vi "Test_peregrine_parameters.vi"() -> ()   [LabVIEW 2019]
panel:
  in  "Value\n(first motor write)":dbl
  out "Decoded value response\n(second motor read)":dbl
  out "Raw value response\n(second motor read)":i32
  out "Key response\n(second motor read)":u32
  out "Decoded value response\n(first motor write)":dbl
  out "Raw value response\n(first motor write)":i32
  out "Key response\n(first motor write)":u32
  out "Decoded value response\n(first motor read)":dbl
  out "Raw value response\n(first motor read)":i32
  out "Key response\n(first motor read)":u32
  in  "Select parameter\n(first motor write)":T1(ring)
  in  "Select parameter\n(first and second for motor read)":T1(ring)
  out "Value response\n(second read)":i32
  out "Key response\n(second read)":u32
  out "Value response\n(first write)":i32
  out "Key response\n(first write)":u32
  in  "Select parameter\n(first write)":T2(ring)
  out "Value response\n(first read)":i32
  out "Key response\n(first read)":u32
  in  "Select parameter\n(first and second read)":T3(ring)
  in  "Address":u8
  in  "COM Port for serial\nconnection. Check device\nmanager.":string
  # "Peregrine test program parameter set and read"
  # "General inputs"
  # "Inputs"
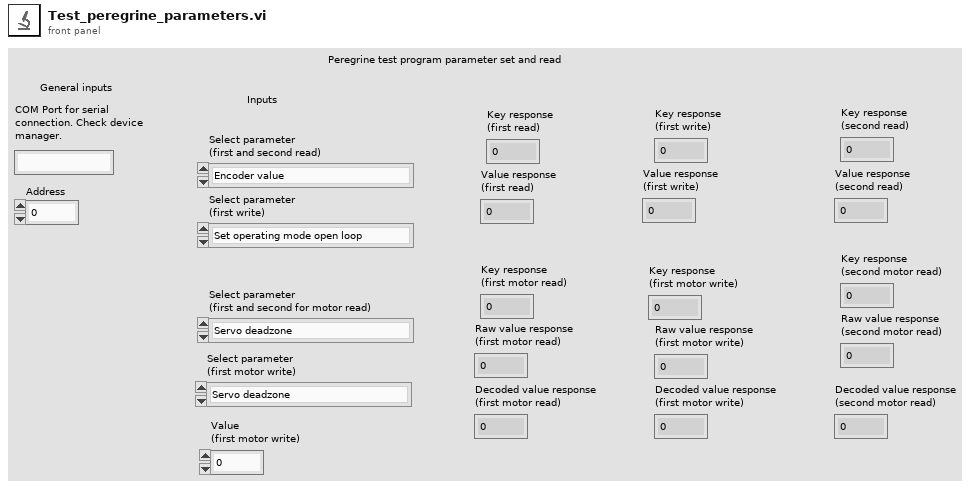
[diagram p1: front panel]
types:
  T1 = enum16{"Servo deadzone", "Position target gain", "Position target P", "Position target D", "V target P", "V target D", "Frequency slew", "Motor direction", "Error gain", "LQR K0", "LQR K1", "LQR B1", "Encoder DIV", "FDIR steprate"}
  T2 = enum16{"Set operating mode open loop", "Set operating mode closed loop", "Set path planning OFF", "Set path planning ON", "Set encoder mode to incremental", "Set encoder mode to absolute", "Set encoder mode to absolute multiturn", "Set microstepping to 8", "Set microstepping to 2", "Set microstepping to 4", "Set microstepping to 16", "Limit switch enabled", "Limit switch disabled", "Limit switch inverted", "Control algorithm PID", "Control algorithm LQR", "Power saving mode", "Power always on"}
  T3 = enum16{"Encoder value", "Operating mode", "Path planning mode", "Encoder mode", "Microstepping mode", "Limit switch mode", "Control mode", "Power save mode", "Read firmware version", "Read driver uptime"}
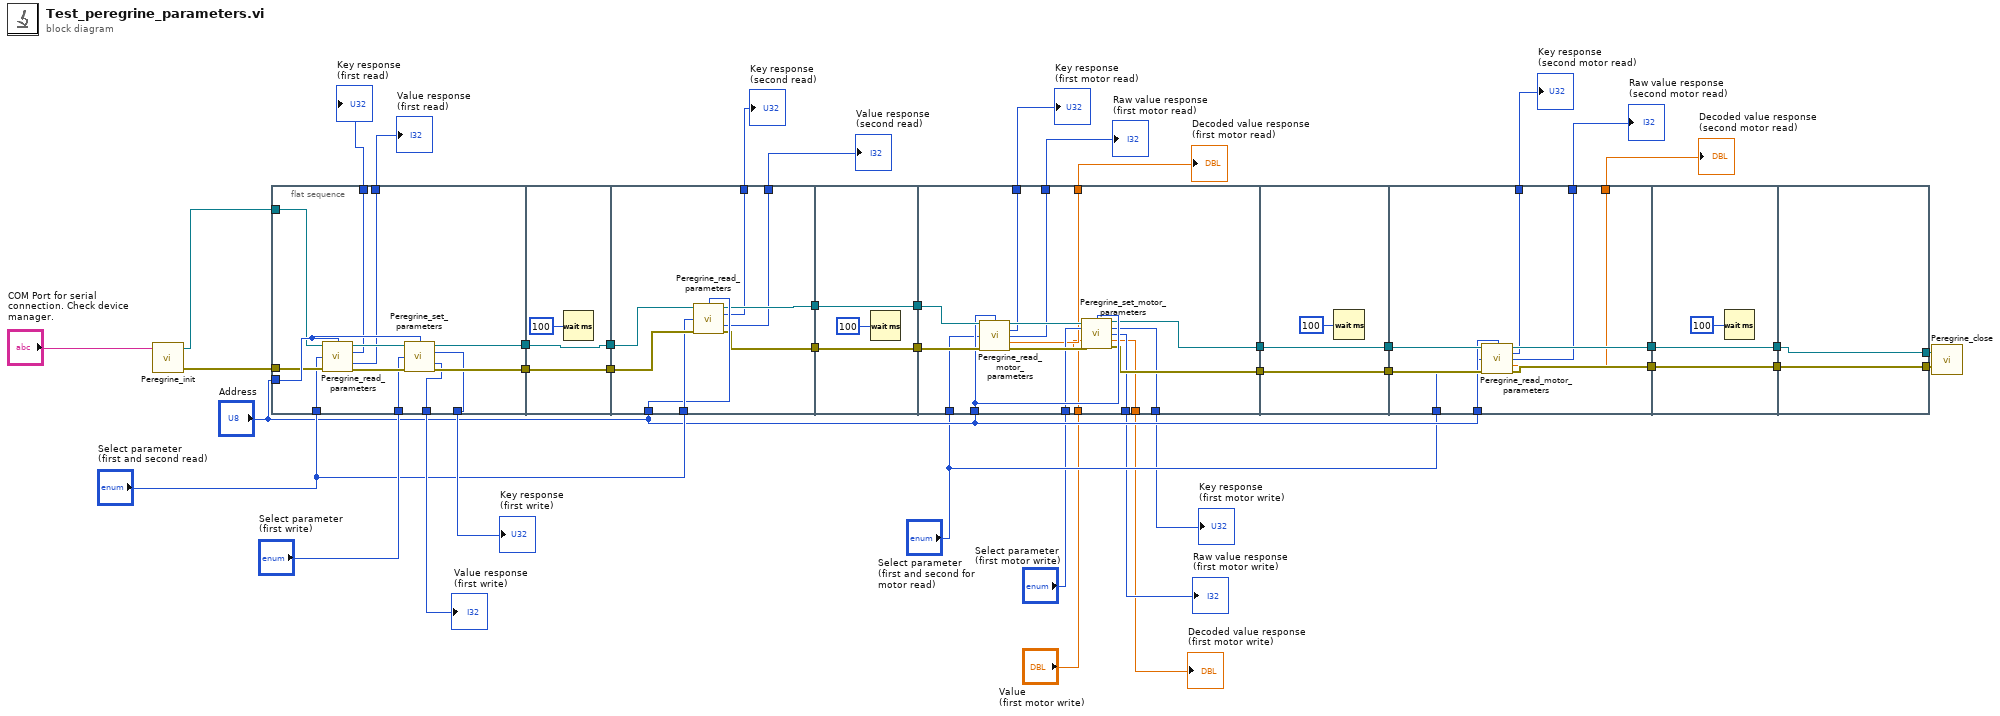
[diagram p0: block diagram]
diagram:
  n1 = call "Peregrine_init.vi"("COM Port for serial\nconnection. Check device\nmanager."="COM Port for serial\nconnection. Check device\nmanager.") -> ("error out"=w40:errorcluster, "Handle out"=w41:refnum<visa-resource-name>)  [unwired: 3 in]
  n2 = flat-sequence {
    tunnel: w41 -> [w54]
    tunnel: "Address" -> [w55]
    tunnel: w40 -> [w53]
    tunnel: "Select parameter\n(first and second read)" -> [w50]
    tunnel: [w49] -> w39
    tunnel: [w48] -> w38
    tunnel: "Select parameter\n(first write)" -> [w47]
    tunnel: [w46] -> w36
    tunnel: [w45] -> w33
    tunnel: [w44] -> w32
    tunnel: [w43] -> w31
    tunnel: w36 -> [w57]
    tunnel: [w57] -> w35
    tunnel: [w56] -> w34
    tunnel: w33 -> [w56]
    tunnel: "Address" -> [w63]
    tunnel: w35 -> [w66]
    tunnel: w34 -> [w65]
    tunnel: "Select parameter\n(first and second read)" -> [w64]
    tunnel: [w62] -> w28
    tunnel: [w61] -> w26
    tunnel: [w60] -> w15
    tunnel: [w59] -> w14
    tunnel: [w68] -> w29
    tunnel: w28 -> [w68]
    tunnel: [w67] -> w27
    tunnel: w26 -> [w67]
    tunnel: w29 -> [w85]
    tunnel: w27 -> [w84]
    tunnel: "Address" -> [w81]
    tunnel: [w80] -> w24
    tunnel: [w79] -> w22
    tunnel: "Select parameter\n(first and second for motor read)" -> [w78]
    tunnel: "Select parameter\n(first motor write)" -> [w77]
    tunnel: [w76] -> w10
    tunnel: [w75] -> w9
    tunnel: [w74] -> w8
    tunnel: [w73] -> w7
    tunnel: [w72] -> w6
    tunnel: [w71] -> w5
    tunnel: "Value\n(first motor write)" -> [w70]
    tunnel: [w87] -> w25
    tunnel: w24 -> [w87]
    tunnel: [w86] -> w23
    tunnel: w22 -> [w86]
    tunnel: w25 -> [w97]
    tunnel: w23 -> [w96]
    tunnel: [w95] -> w20
    tunnel: [w94] -> w18
    tunnel: "Address" -> [w93]
    tunnel: "Select parameter\n(first and second for motor read)" -> [w92]
    tunnel: [w91] -> w4
    tunnel: [w90] -> w3
    tunnel: [w89] -> w2
    tunnel: [w99] -> w21
    tunnel: w20 -> [w99]
    tunnel: [w98] -> w19
    tunnel: w18 -> [w98]
    tunnel: w21 -> [w102]
    tunnel: w19 -> [w101]
    tunnel: [w102] -> w17
    tunnel: [w101] -> w16
    frame #0 {
      n3 = call "Peregrine_read_parameters.vi"("Handle in"=w54, "Address"=w55, "Select parameter"=w50, "error"=w53) -> ("Handle out"=w51:refnum<visa-resource-name>, "Key response"=w49:u32, "Value response"=w48:i32, "error out"=w52:errorcluster)  [unwired: 8 in]
      n4 = call "Peregrine_set_parameters.vi"("Handle in"=w51, "Address"=w55, "Select parameter"=w47, "error"=w52) -> ("Handle out"=w46:refnum<visa-resource-name>, "Key response"=w44:u32, "Value response"=w43:i32, "error out"=w45:errorcluster)  [unwired: 8 in]
    }
    frame #1 {
      n5 = Wait (ms)(milliseconds to wait=u32 100) -> ()  [unwired: 1 out]
    }
    frame #2 {
      n6 = call "Peregrine_read_parameters.vi"("Handle in"=w66, "Address"=w63, "Select parameter"=w64, "error"=w65) -> ("Handle out"=w62:refnum<visa-resource-name>, "Key response"=w60:u32, "Value response"=w59:i32, "error out"=w61:errorcluster)  [unwired: 8 in]
    }
    frame #3 {
      n7 = Wait (ms)(milliseconds to wait=u32 100) -> ()  [unwired: 1 out]
    }
    frame #4 {
      n8 = call "Peregrine_read_motor_parameters.vi"("Handle in"=w85, "Address"=w81, "Select parameter"=w78, "error"=w84) -> ("Handle out"=w82:refnum<visa-resource-name>, "Key response"=w76:u32, "Raw value response"=w75:i32, "Decoded value response"=w74:dbl, "error out"=w83:errorcluster)  [unwired: 7 in]
      n9 = call "Peregrine_set_motor_parameters.vi"("Handle in"=w82, "Address"=w81, "Select parameter"=w77, "Value"=w70, "error"=w83) -> ("Handle out"=w80:refnum<visa-resource-name>, "Key response"=w73:u32, "Raw value response"=w72:i32, "Decoded value response"=w71:dbl, "error out"=w79:errorcluster)  [unwired: 6 in]
    }
    frame #5 {
      n10 = Wait (ms)(milliseconds to wait=u32 100) -> ()  [unwired: 1 out]
    }
    frame #6 {
      n11 = call "Peregrine_read_motor_parameters.vi"("Handle in"=w97, "Address"=w93, "Select parameter"=w92, "error"=w96) -> ("Handle out"=w95:refnum<visa-resource-name>, "Key response"=w91:u32, "Raw value response"=w90:i32, "Decoded value response"=w89:dbl, "error out"=w94:errorcluster)  [unwired: 7 in]
    }
    frame #7 {
      n12 = Wait (ms)(milliseconds to wait=u32 100) -> ()  [unwired: 1 out]
    }
    frame #8 {
    }
  }
  n13 = call "Peregrine_close.vi"("error in (no error)"=w16, "Handle in"=w17) -> ()  [unwired: 1 in, 1 out]
  "Key response\n(first read)" <- w39
  "Value response\n(first read)" <- w38
  "Key response\n(first write)" <- w32
  "Value response\n(first write)" <- w31
  "Key response\n(second read)" <- w15
  "Value response\n(second read)" <- w14
  "Key response\n(first motor read)" <- w10
  "Raw value response\n(first motor read)" <- w9
  "Decoded value response\n(first motor read)" <- w8
  "Key response\n(first motor write)" <- w7
  "Raw value response\n(first motor write)" <- w6
  "Decoded value response\n(first motor write)" <- w5
  "Key response\n(second motor read)" <- w4
  "Raw value response\n(second motor read)" <- w3
  "Decoded value response\n(second motor read)" <- w2
